vi "MB Ethernet String to Modbus Data Unit.vi"(8 "error in (no error)":errorcluster, 11 "data":u8[](array[numeric])) -> (0 "error out":errorcluster, 1 "Exception Code":u8 format="%.0x", 3 "Modbus Data Unit":T1={"function"=1, "Data"=[]} {"function" items=["Read Discrete Inputs"=2, "Read Coils"=1, "Write Single Coil"=5, "Write Multiple Coils"=15, "Read Input Register"=4, "Read Holding Registers"=3, "Write Single Register"=6, "Write Multiple Registers"=16, "Read/Write Multiple Registers"=23, "Mask Write Register"=22, "Read FIFO Queue"=24, "Read File Record"=20, "Write File Record"=21, "Read Exception Status"=7, "Diagnostic"=8, "Get Com Event Counter"=11, "Get Com Event Log"=12, "Report Slave ID"=17, "Read Device Identification"=43]; "Data" format="%.0x"})   [LabVIEW 2019, in "NI_modbus_upd.lvlib"]
uses:
  NI_modbus_upd.lvlib
  Ctl/MB Modbus Data Unit.ctl
  Modbus Data Unit (PDU)/Function.ctl
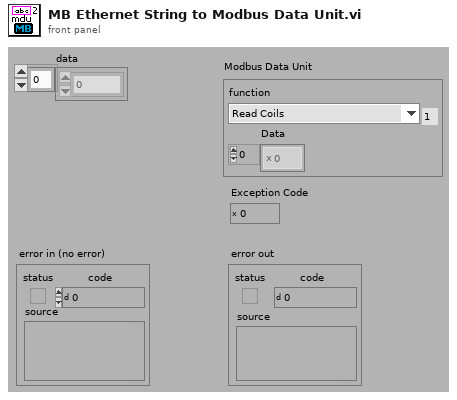
[diagram p1: front panel]
types:
  T1 = typedef "NI_modbus_upd.lvlib/MB Modbus Data Unit.ctl" = cluster{"function":T2, "Data":u8[]}
  T2 = typedef "NI_modbus_upd.lvlib/Function.ctl" = u8
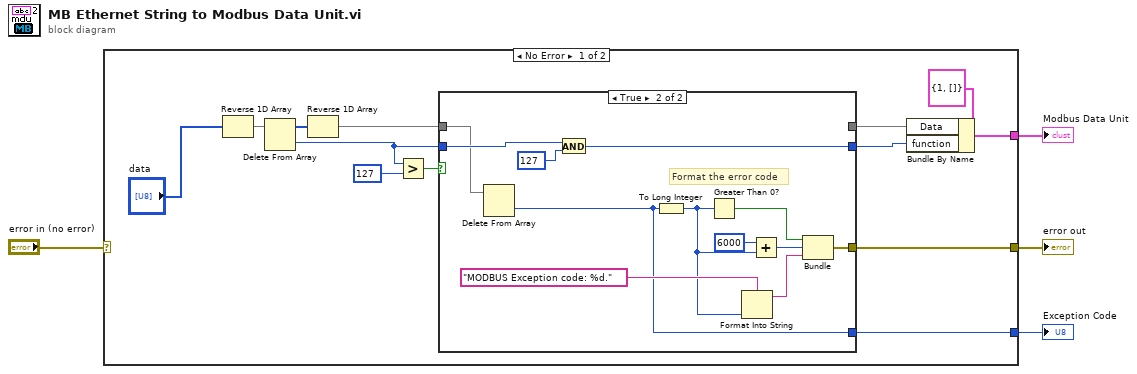
[diagram p0: block diagram]
diagram:
  n1 = case shown="No Error" "error in (no error)" {
    selector: "error in (no error)" -> [_ w32]
    tunnel: [w14 _] -> w4
    tunnel: [w13 w32] -> w2
    tunnel: [w15 _] -> w1
    frame No Error {
      n2 = Reverse 1D Array(array="data") -> (reversed array=w12:u8[])
      n3 = Delete From Array(array=w12) -> (deleted portion=w9:u8, array with subset deleted=w11:u8[])  [unwired: 2 in]
      n4 = Reverse 1D Array(array=w11) -> (reversed array=w10:u8[])
      n5 = Greater?(x=w9, y=u8 127) -> (0:w16:bool)
      n6 = case shown="True" w16 {
        tunnel: [w18 _] -> w6
        tunnel: w9 -> [w19 w30]
        tunnel: [w19 w29] -> w7
        tunnel: [_ w20] -> w14
        tunnel: [_ w22] -> w13
        tunnel: w10 -> [w18 w21]
        frame False {
        }
        frame True {
          # "Format the error code"
          n7 = Delete From Array(array=w21) -> (deleted portion=w20:u8)  [unwired: 2 in, 1 out]
          n8 = And(x=w30, y=u8 127) -> (x .and. y?=w29:u8)
          n9 = To Long Integer(number=w20) -> (32bit integer=w23:i32)
          n10 = Greater Than 0?(x=w23) -> (x > 0?=w28:bool)
          n11 = Format Into String(format string="MODBUS Exception code: %d.", w23) -> (resulting string=w27:string)  [unwired: 2 in, 1 out]
          n12 = Add(x=6000 ("New Error Code"), y=w23) -> (x+y=w25:i32)
          n13 = Bundle(w28, w25, w27) -> (w22:errorcluster)  [unwired: 1 in]
        }
      }
      n14 = Bundle By Name(cluster=T1 {"function"=1, "Data"=[]} ("Modbus Data Unit"), "Data"=w6, "function"=w7) -> (w15:T1)
    }
    frame Error {
    }
  }
  "error out" <- w2
  "Exception Code" <- w4
  "Modbus Data Unit" <- w1
